vi "DOE Capacity Measurment.vi"(8 "error in (no error)":errorcluster, 10 "Config State":T1, 11 "DOE Capacity Measurments":T2) -> (0 "error out":errorcluster, 3 "DOE Capacity Measurments Output":T2)   [LabVIEW 2016]
doc: "This VI allows the user to input the capacity measurments if required"
uses:
  Type Definitions/DOE Capacity Measurments.ctl
  Utility/Custom Pallet Controls/Custom Pallet Forward.ctl
  Utility/Save File/File Setup (Public)/Type Definition/Save File DOE Configuration State.ctl
  Utility/Save File/File Setup.lvlib
panel:
  in  "File Setup OK":T3
  out "Test Date:DOE Cap":timestamp caption="Test Date:"
  # "DOE Capacity Measurements Per 10 CFR 430 Appendix J1"
  # "Model Number"
  # "Serial Number"
  # "Lab Number"
  # "Weight of Water (Lbs)"
  # "Measured Temp (F)"
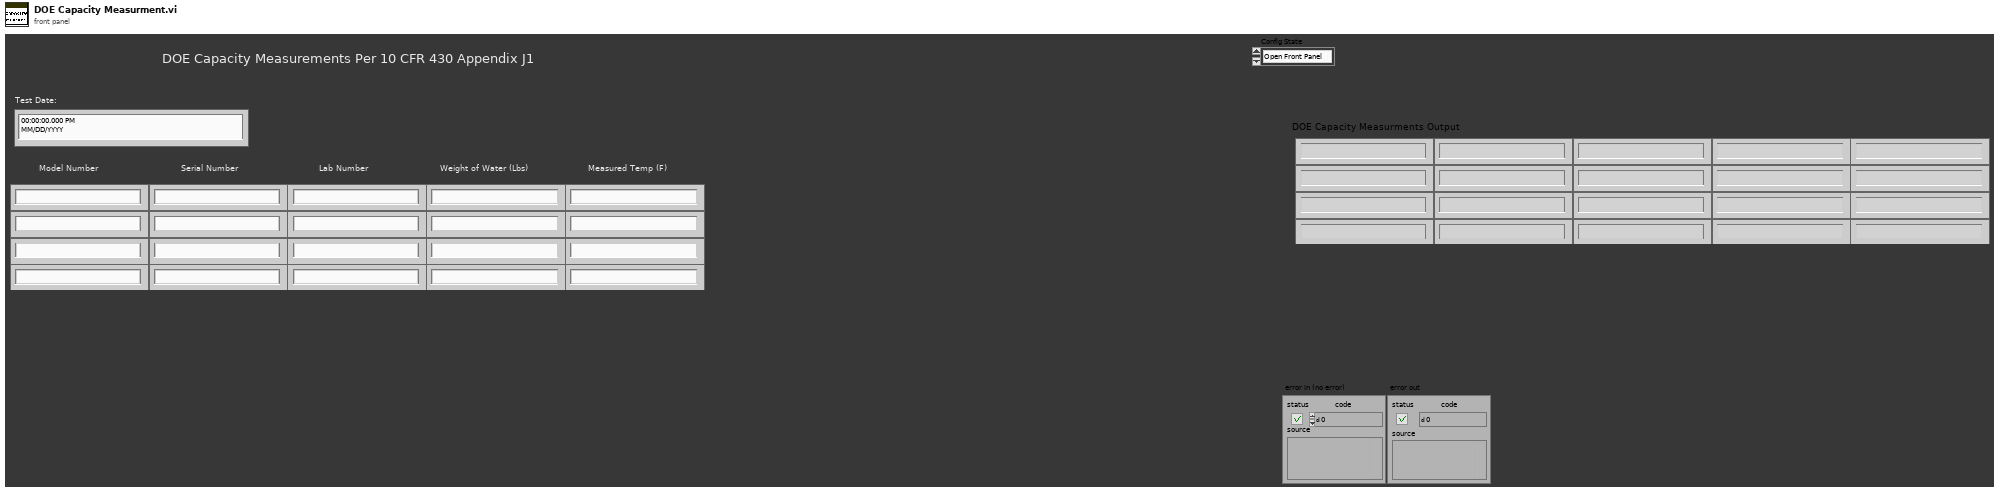
[diagram p1: front panel]
types:
  T1 = typedef "File Setup.lvlib/Save File DOE Configuration State.ctl" = enum16{"Open Front Panel", "Load Config"}
  T2 = typedef "DOE Capacity Measurments.ctl" = cluster{"Weight 1":dbl, "Model Number 1":string, "Temp 1":dbl, "Serial Number 1":string, "Lab Number 1":string, "Lab Number 2":string, "Serial Number 2":string, "Temp 2":dbl, "Model Number 2":string, "Weight 2":dbl, "Lab Number 3":string, "Serial Number 3":string, "Temp 3":dbl, "Model Number 3":string, "Weight 3":dbl, "Lab Number 4":string, "Serial Number 4":string, "Temp 4":dbl, "Model Number 4":string, "Weight 4":dbl, "Capacity Measurment Output String":string[][]}
  T3 = typedef "Custom Pallet Forward.ctl" = bool
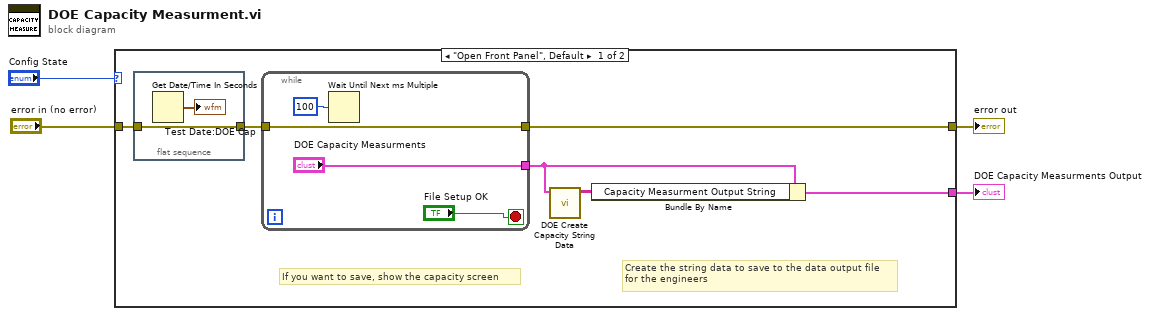
[diagram p0: block diagram]
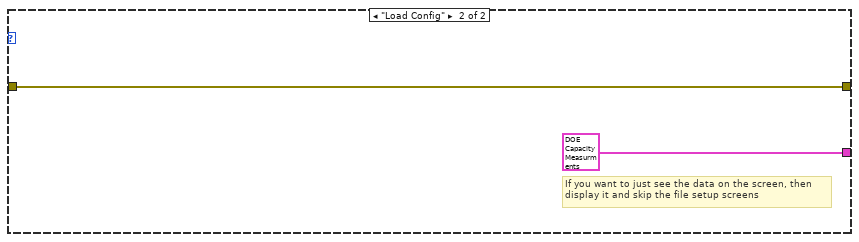
[diagram p2: hidden frame]
diagram:
  n1 = case shown="\"Open Front Panel\", Default" "Config State" {
    tunnel: "error in (no error)" -> [w10 w18]
    tunnel: [w8 w18] -> w3
    tunnel: [w6 T2 {"Weight 1"=0.0, "Model Number 1"="", "Temp 1"=0.0, "Serial Number 1"="", "Lab Number 1"="", "Lab Number 2"="", "Serial Number 2"="", "Temp 2"=0.0, "Model Number 2"="", "Weight 2"=0.0, "Lab Number 3"="", "Serial Number 3"="", "Temp 3"=0.0, "Model Number 3"="", "Weight 3"=0.0, "Lab Number 4"="", "Serial Number 4"="", "Temp 4"=0.0, "Model Number 4"="", "Weight 4"=0.0, "Capacity Measurment Output String"=[]} ("DOE Capacity Measurments")] -> w2
    frame "Open Front Panel", Default {
      # "Create the string data to save to the data output file\nfor the engineers"
      # "If you want to save, show the capacity screen"
      n2 = flat-sequence {
        tunnel: w10 -> [w11]
        tunnel: [w11] -> w9
        frame #0 {
          n3 = Get Date/Time In Seconds() -> (seconds since 1Jan1904=→"Test Date:DOE Cap":timestamp)
        }
      }
      n4 = while {
        tunnel: w9 -> [w16]
        tunnel: [w16] -> w8
        tunnel: ["DOE Capacity Measurments"] -> w7
        stop <- "File Setup OK" stop-if-true
        n5 = Wait Until Next ms Multiple(millisecond multiple=u32 100) -> ()  [unwired: 1 out]
      }
      n6 = call "DOE Create Capacity String Data.vi"("DOE Capacity Measurments"=w7) -> ("Capacity Measurement String Output"=w5:string[][])  [unwired: 10 in]
      n7 = Bundle By Name(cluster=w7, "Capacity Measurment Output String"=w5) -> (w6:T2)
    }
    frame "Load Config" {
      # "If you want to just see the data on the screen, then\ndisplay it and skip the file setup screens"
    }
  }
  "error out" <- w3
  "DOE Capacity Measurments Output" <- w2
